vi "Get Integer Increment.vi"(8 "error in (no error)":errorcluster, 11 "Camera in":refnum<class "Camera.lvclass">) -> (0 "error out":errorcluster, 2 "Increment":i32, 3 "Camera":refnum<class "Camera.lvclass">)   [LabVIEW 2020]
uses:
  Camera.lvclass
  Camera.lvclass/Camera.ctl
  bin/gindustrialcam_32-1.dll
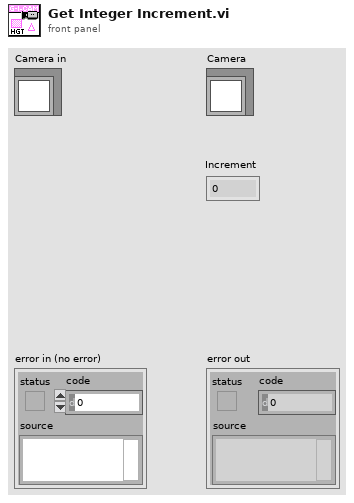
[diagram p1: front panel]
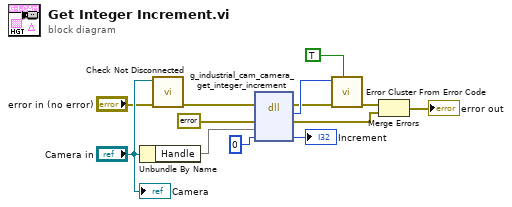
[diagram p0: block diagram]
diagram:
  n1 = Unbundle By Name("Camera in") -> ("Handle"=w8)
  n2 = call "Check Not Disconnected.vi"("error in (no error)"="error in (no error)", "Camera in"="Camera in") -> ("error out"=w9:errorcluster)  [unwired: 9 in]
  n3 = dll-call lib="C:/serenial/lib/g-industrial-camera/LabVIEW/g_industrial_cam/bin/gindustrialcam_*-1.*" fn="g_industrial_cam_camera_get_integer_increment"(error in=w9, "err"=errorcluster {"status"=FALSE, "code"=0, "source"=""} ("error constant"), "edvr"=w8, "increment"=0 ("Value In")) -> (error out=w2:errorcluster, "Mg_Error"=w3:i32, "err"=w5:errorcluster, "increment"=→"Increment":i32)  [unwired: 3 in, 1 out]
  n4 = call <vilib>:"Error Cluster From Error Code.vi"("show call chain? (False)"=TRUE, "error in (no error)"=w2, "error code (0)"=w3) -> ("error out"=w4:errorcluster)  [unwired: 6 in]
  n5 = Merge Errors(w4, w5) -> (→"error out":errorcluster)
  "Camera" <- "Camera in"
